vi "Math-NaN Mean (2D).vi"(1 "Array":dbl[][](array[numeric])) -> (0 "NaN Mean":dbl[](array[numeric]))   [LabVIEW 2015]
uses:
  <vilib>/Analysis/baseanly.llb/Mean (DBL).vi
  <vilib>/Analysis/NI_AALBase.lvlib
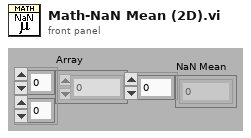
[diagram p1: front panel]
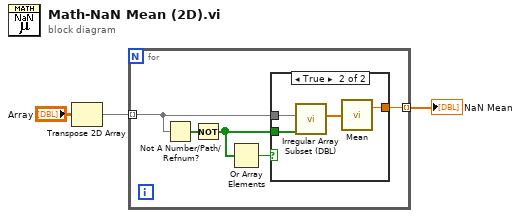
[diagram p0: block diagram]
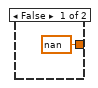
[diagram p2: hidden frame]
diagram:
  n1 = Transpose 2D Array(2D array="Array") -> (transposed array=w1:dbl[][])
  n2 = for {
    tunnel: [w8] -> w3 mode=indexing
    tunnel: w1 -> [w4] mode=indexing
    n3 = Not A Number/Path/Refnum?(number/path/refnum=w4) -> (NaN/Path/Refnum?=w7:bool[])
    n4 = Not(x=w7) -> (.not. x?=w6:bool[])
    n5 = Or Array Elements(Boolean array=w6) -> (logical OR=w5:bool)
    n6 = case shown="True" w5 {
      tunnel: [nan ("mean") w13] -> w8
      tunnel: w4 -> [_ w12]
      tunnel: w6 -> [_ w10]
      frame False {
      }
      frame True {
        n7 = call "Irregular Array Subset (DBL).vi"("Mask"=w10, "Array"=w12) -> ("Array Subset"=w11:dbl[])  [unwired: 8 in, 1 out]
        n8 = call-poly <vilib>:"Mean.vi"("X"=w11) -> ("mean"=w13:dbl)  [unwired: 1 out]
      }
    }
  }
  "NaN Mean" <- w3
